vi "Launch CS++StartActor.vi"() -> ()   [LabVIEW 2013]
doc: "Launch CS++StartActor.\n\nUse command line parameters in case of Run Time System.\nDB=\"DB Connection String\"; Default:\"ApplicationName.ini\"\nFactory=\"Path to desired Factory class\"; Default: \"emptyString\" use CS++Factory \nStartActor=\"Name of desired start actor\"; Default: \"CS++StartActor\""
uses:
  Classes/CS++BaseClasses/Factory/CS++Factory.lvclass
  Classes/CS++BaseClasses/Factory/CS++Factory.lvclass/CS++Factory.ctl
  <vilib>/ActorFramework/Message Queue/Message Queue.lvclass/Message Queue.ctl
  <vilib>/ActorFramework/Actor/Actor.lvclass
  <vilib>/ActorFramework/Message Queue/Message Queue.lvclass
panel:
  in  "Type":T1={"DB Connection String"="C:\\User\\Brand\\Git\\CSPP\\Examples\\CS++Example.ini", "Start Actor"="CS++StartActor", "CS++Factory"=path ""}
  in  "CS++Factory":path
  in  "Start Actor":string="CS++StartActor"
  out "Attributes found?":bool=TRUE
  in  "DB Connection String":string="C:\\User\\Brand\\Git\\CSPP\\Examples\\CS++Example.ini"
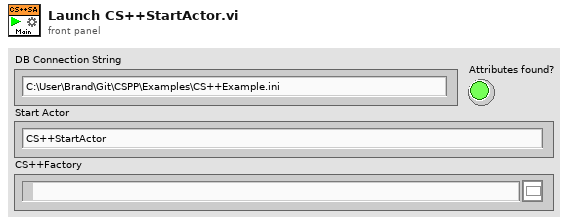
[diagram p1: front panel]
types:
  T1 = cluster{"DB Connection String":string, "Start Actor":string, "CS++Factory":path}
  T2 = enum32{"invalid app kind", "Development System", "Run Time System", "Student Edition", "Embedded LabVIEW", "Evaluation", "Custom"}
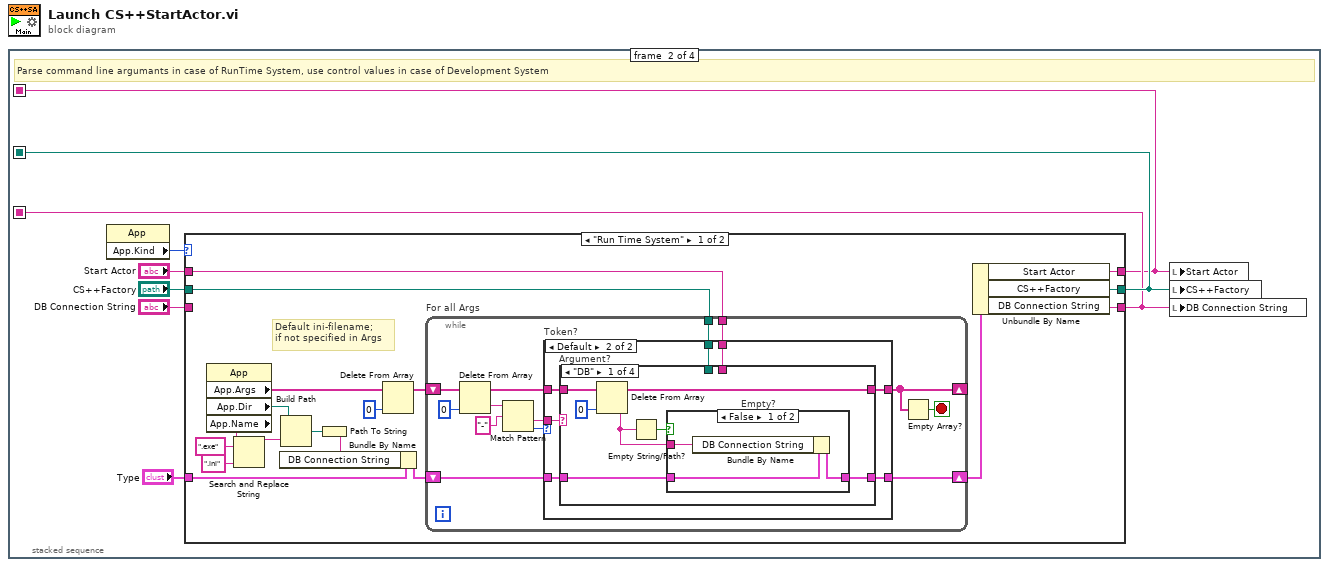
[diagram p0: block diagram]
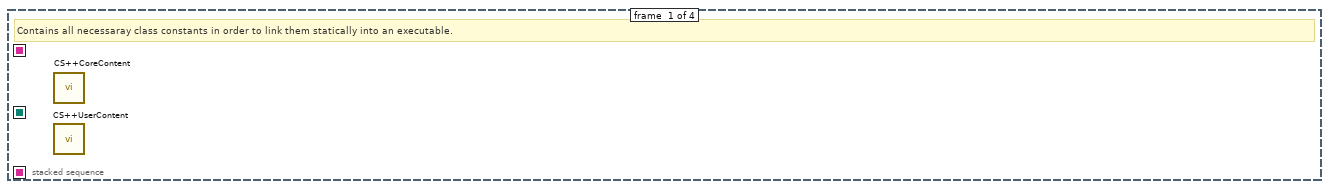
[diagram p2: hidden frame]
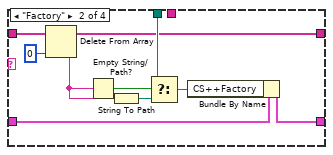
[diagram p5: hidden frame]
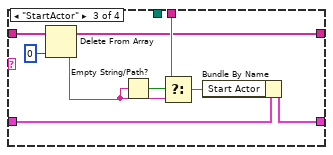
[diagram p6: hidden frame]
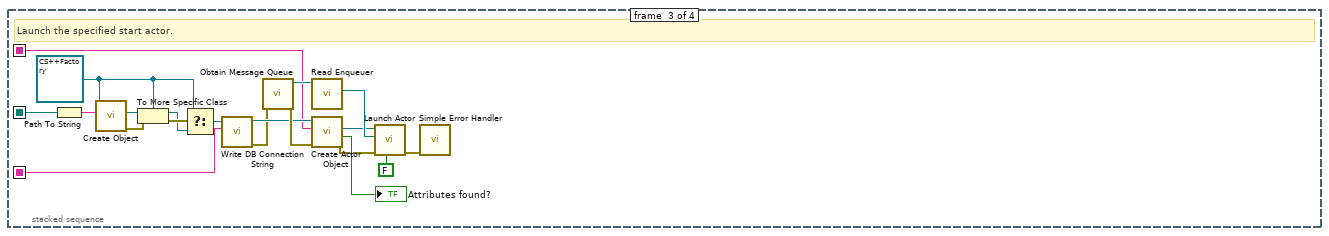
[diagram p9: hidden frame]
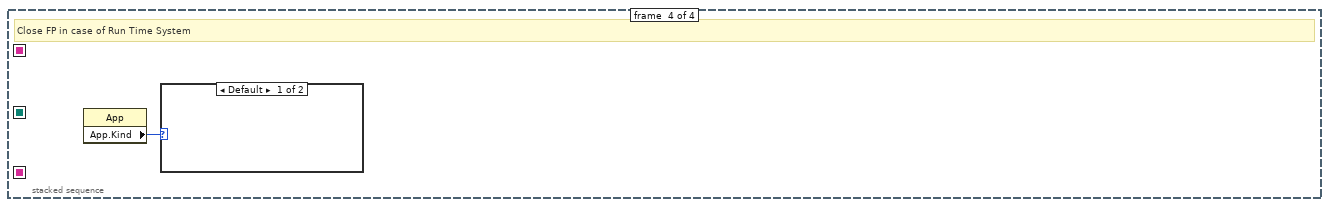
[diagram p10: hidden frame]
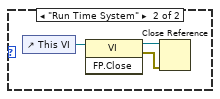
[diagram p11: hidden frame]
diagram:
  n1 = stacked-sequence {
    seq-local: [_ w2 _ _] -> [_ _ w90 _]
    seq-local: [_ w3 _ _] -> [_ _ w88 _]
    seq-local: [_ w1 _ _] -> [_ _ w89 _]
    frame #0 {
      # "Contains all necessaray class constants in order to link them statically into an executable."
      n2 = call "CS++CoreContent.vi"() -> ()  [unwired: 12 in]
      n3 = call "CS++UserContent.vi"() -> ()  [unwired: 12 in]
    }
    frame #1 {
      # "Parse command line argumants in case of RunTime System, use control values in case of Development System"
      n4 = property class="App"() -> ("App.Kind"=w8:T2)  [unwired: 2 in, 2 out]
      n5 = case shown="\"Run Time System\"" w8 {
        tunnel: [w16 w83] -> w1
        tunnel: "Start Actor" -> [w19 w83]
        tunnel: [w15 w82] -> w3
        tunnel: "CS++Factory" -> [w18 w82]
        tunnel: [w14 w81] -> w2
        tunnel: "DB Connection String" -> [_ w81]
        tunnel: "Type" -> [w12 _]
        frame "Run Time System" {
          # "Default ini-filename;\nif not specified in Args"
          n6 = property class="App"() -> ("App.Args"=w10:string[], "App.Dir"=w22:path, "App.Name"=w21:string)  [unwired: 2 in, 2 out]
          n7 = Search and Replace String(input string=w21, search string=".exe", replace string=".ini" ("replace string (\"\")")) -> (result string=w25:string)  [unwired: 5 in, 3 out]
          n8 = Build Path(base path=w22, name or relative path=w25) -> (appended path=w26:path)
          n9 = Path To String(path=w26) -> (string=w9:string)
          n10 = Bundle By Name(cluster=w12, "DB Connection String"=w9) -> (w11:T1)
          n11 = Delete From Array(array=w10, index=0) -> (array with subset deleted=w20:string[])  [unwired: 1 in, 1 out]
          n12 = while "For all Args" {
            shift-right: [w38] -> w17
            shift-left: w11 -> [w39]
            tunnel: w19 -> [w37]
            tunnel: w18 -> [w36]
            shift-right: [w31] -> _
            shift-left: w20 -> [w35]
            stop <- w32 stop-if-true
            n13 = Delete From Array(array=w35, index=0) -> (deleted portion=w30:string, array with subset deleted=w34:string[])  [unwired: 1 in]
            n14 = Match Pattern(string=w30, regular expression="-" ("search string/char (-)")) -> (after substring=w28:string, offset past match=w27:i32)  [unwired: 1 in, 2 out]
            n15 = case "Token?" shown="Default" w27 {
              tunnel: w39 -> [w40 w48]
              tunnel: [w40 w47] -> w38
              tunnel: w37 -> [_ w46]
              tunnel: w36 -> [_ w45]
              tunnel: w28 -> [_ w44]
              tunnel: w34 -> [w41 w43]
              tunnel: [w41 w42] -> w31
              frame -1 {
              }
              frame Default {
                n16 = case "Argument?" shown="\"DB\"" w44 {
                  tunnel: w48 -> [w55 w69 w78 w80]
                  tunnel: [w54 w68 w77 w80] -> w47
                  tunnel: w46 -> [_ _ w74 _]
                  tunnel: w45 -> [_ w65 _ _]
                  tunnel: [w52 w61 w71 w79] -> w42
                  tunnel: w43 -> [w53 w62 w72 w79]
                  frame "DB" {
                    n17 = Delete From Array(array=w53, index=0) -> (deleted portion=w50:string, array with subset deleted=w52:string[])  [unwired: 1 in]
                    n18 = Empty String/Path?(string/path=w50) -> (empty?=w49:bool)
                    n19 = case "Empty?" shown="False" w49 {
                      tunnel: w55 -> [w58 w59]
                      tunnel: [w57 w59] -> w54
                      tunnel: w50 -> [w56 _]
                      frame False {
                        n20 = Bundle By Name(cluster=w58, "DB Connection String"=w56) -> (w57:T1)
                      }
                      frame True {
                      }
                    }
                  }
                  frame "Factory" {
                    n21 = Delete From Array(array=w62, index=0) -> (deleted portion=w60:string, array with subset deleted=w61:string[])  [unwired: 1 in]
                    n22 = Empty String/Path?(string/path=w60) -> (empty?=w67:bool)
                    n23 = String To Path(string=w60) -> (path=w64:path)
                    n24 = Select(t=w65, s=w67, f=w64) -> (s? t:f=w66:path)
                    n25 = Bundle By Name(cluster=w69, "CS++Factory"=w66) -> (w68:T1)
                  }
                  frame "StartActor" {
                    n26 = Delete From Array(array=w72, index=0) -> (deleted portion=w70:string, array with subset deleted=w71:string[])  [unwired: 1 in]
                    n27 = Empty String/Path?(string/path=w70) -> (empty?=w76:bool)
                    n28 = Select(t=w74, s=w76, f=w70) -> (s? t:f=w75:string)
                    n29 = Bundle By Name(cluster=w78, "Start Actor"=w75) -> (w77:T1)
                  }
                  frame Default {
                  }
                }
              }
            }
            n30 = Empty Array?(array=w31) -> (empty?=w32:bool)
          }
          n31 = Unbundle By Name(w17) -> ("Start Actor"=w16:string, "CS++Factory"=w15:path, "DB Connection String"=w14:string)
        }
        frame "Development System", Default {
        }
      }
      n32 = local write "Start Actor"(w1) -> ()
      n33 = local write "CS++Factory"(w3) -> ()
      n34 = local write "DB Connection String"(w2) -> ()
    }
    frame #2 {
      w86 = refnum<class "CS++Factory.lvclass"> refnum ("CS++BaseClasses.lvlib:CS++Factory.lvclass")
      # "Launch the specified start actor."
      n35 = Path To String(path=w88) -> (string=w87:string)
      n36 = call "Create Object.vi"("Object Name"=w87, "CS++Factory in"=w86) -> ("error out"=w84:errorcluster, "LabVIEW Object"=w85:refnum<class>)  [unwired: 6 in, 2 out]
      n37 = To More Specific Class(target class=w86, reference=w85, error in=w84) -> (specific class reference=w94:refnum<class "CS++Factory.lvclass">, error out=w95:errorcluster)
      n38 = Select(t=w86, s=w95, f=w94) -> (s? t:f=w93:refnum<class "CS++Factory.lvclass">)
      n39 = call "Write DB Connection String.vi"("DB Connection String"=w90, "CS++Factory in"=w93) -> ("error out"=w92:errorcluster, "CS++Factory out"=w98:refnum<class "CS++Factory.lvclass">)  [unwired: 8 in]
      n40 = call <vilib>:"Obtain Message Queue.vi"("error in (no error)"=w92) -> ("error out"=w102:errorcluster, "Message Queue"=w103:refnum<class "Message Queue.lvclass">)  [unwired: 9 in]
      n41 = call <vilib>:"Read Enqueuer.vi"("Message Queue"=w103) -> ("Message Enqueuer"=w101:refnum<class "Message Enqueuer.lvclass">)  [unwired: 10 in]
      n42 = call "Create Actor Object.vi"("error in (no error)"=w102, "Object Name"=w89, "CS++Factory in"=w98) -> ("error out"=w96:errorcluster, "Attributes found?"=→"Attributes found?":bool, "C++BaseActor"=w97:refnum<class "CS++BaseActor.lvclass">)  [unwired: 5 in, 1 out]
      n43 = call <vilib>:"Launch Actor.vi"("Open Actor Core front panel? (F)"=FALSE, "error in (no error)"=w96, "Actor-to-Caller Enqueuer"=w101, "Actor"=w97) -> ("error out"=w91:errorcluster)  [unwired: 6 in, 1 out]
      n44 = call <vilib>:"Simple Error Handler.vi"("error in (no error)"=w91) -> ()  [unwired: 4 in, 5 out]
    }
    frame #3 {
      # "Close FP in case of Run Time System"
      n45 = property class="App"() -> ("App.Kind"=w104:T2)  [unwired: 2 in, 2 out]
      n46 = case shown="Default" w104 {
        frame Default {
        }
        frame "Run Time System" {
          n47 = control-ref of="This VI"() -> (w107:refnum<vi>)
          n48 = invoke class="VI" method="FP.Close"(reference=w107) -> (reference out=w106:refnum<vi>, error out=w105:errorcluster)  [unwired: 2 in, 1 out]
          n49 = Close Reference(reference=w106, error in (no error)=w105) -> ()  [unwired: 1 out]
        }
      }
    }
  }
